vi "Untitled 13.vi"   [LabVIEW 2016]
uses:
  Motor controllers.vi
  Set control mode.vi
  Set Speed or Torque.vi
  <vilib>/CANopenLib/CANOPEN.llb/CANopen SDO Create.vi
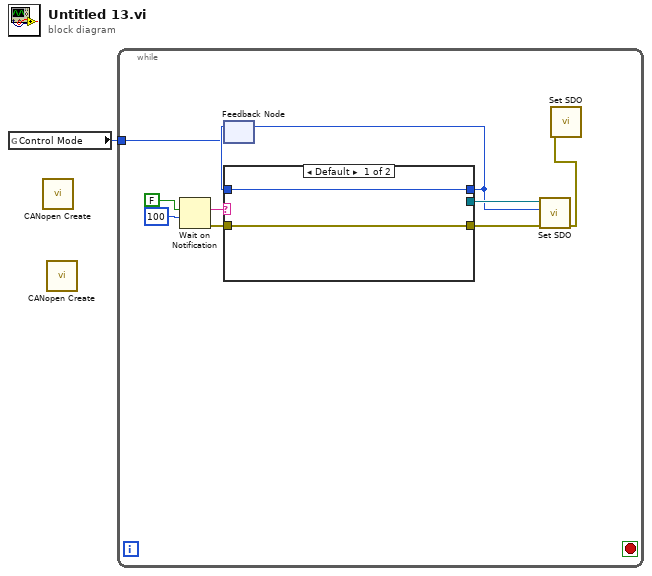
[diagram p0: block diagram]
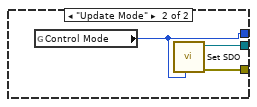
[diagram p2: hidden frame]
diagram:
  n1 = global read "Motor controllers.vi" "Control Mode"() -> (w1:u8)
  n2 = call-poly <vilib>:"CANopen Create.vi"() -> ()  [unwired: 9 in, 3 out]
  n3 = call-poly <vilib>:"CANopen Create.vi"() -> ()  [unwired: 9 in, 3 out]
  n4 = while {
    tunnel: w1 -> [w6]
    stop <- _ stop-if-true
    n5 = Wait on Notification(ignore previous (F)=FALSE, timeout in ms (-1)=100) -> (notification=w8:string, error out=w9:errorcluster)  [unwired: 2 in, 2 out]
    n6 = feedback #1(w6) -> (w7:u8)
    n7 = case shown="Default" w8 {
      tunnel: w9 -> [w12 _]
      tunnel: w7 -> [w13 _]
      tunnel: [w13 w16] -> w3
      tunnel: [w12 w15] -> w5
      tunnel: [_ w14] -> w4
      frame Default {
      }
      frame "Update Mode" {
        n8 = global read "Motor controllers.vi" "Control Mode"() -> (w16:u8)
        n9 = call-poly "Set SDO.vi"("Control Mode"=w16) -> ("error out"=w15:errorcluster, "SDO object out"=w14:refnum<k20>)  [unwired: 8 in, 1 out]
      }
    }
    n10 = feedback-in #1(w3) -> ()
    n11 = call-poly "Set SDO.vi"("error in (no error)"=w5, "Torque"=w3, "SDO object in"=w4) -> ("error out"=w2:errorcluster)  [unwired: 6 in, 2 out]
    n12 = call-poly "Set SDO.vi"("error in (no error)"=w2) -> ()  [unwired: 8 in, 3 out]
  }
